vi "Receiver.vi"() -> ()   [LabVIEW 2015]
uses:
  <vilib>/addons/Modulation/Analog/support/mod_Set Error Source.vi
  <vilib>/addons/Modulation/Analog/support/Validators/mod_Fractional Resample Validate.vi
  <vilib>/addons/Modulation/Analog/support/Validators/mod_Check Flush State.vi
  <vilib>/addons/Modulation/Analog/support/mod_FractionalResampler.vi
  <vilib>/addons/Modulation/Analog/support/mod_Integer Rate Interpolation.vi
  <vilib>/addons/Modulation/Analog/support/Validators/mod_Validate Complex Waveform.vi
  <vilib>/addons/Modulation/Analog/support/mod_PerformResampling.vi
  <vilib>/addons/Modulation/Analog/support/Validators/mod_WFErrorHandler.vi
  <vilib>/addons/Modulation/Digital/General/MT Generate PSK System Parameters(M).vi
  <vilib>/addons/Modulation/Digital/Support/Common/Validators/mod_Generate Filter Coefficients Validate.vi
  <vilib>/addons/Modulation/Digital/General/subVIs/mod_Generate Filter Coefficients.vi
  <instrlib>/niUSRP/niUSRP Fetch Rx Data (CDB Cluster).vi
  <vilib>/Utility/error.llb/Error Cluster From Error Code.vi
  <vilib>/addons/Modulation/Analog/support/mod_Resampling Factors.vi
  <vilib>/addons/Modulation/Analog/support/mod_ResamplingFilter.vi
  <vilib>/addons/Modulation/Analog/support/mod_Generate Integer Interpolation Filter.vi
  <vilib>/addons/Modulation/niDMT.lvlib
  <vilib>/addons/Modulation/niAMT.lvlib
panel:
  in  "stop":bool
  in  "Reset":bool=TRUE caption="Reset\nDemodulator?"
  out "measurements":T1={"frequency offset (Hz)"=-11.93165072236316, "frequency drift (Hz)"=0.08770196207837619, "phase offset (deg)"=52.673364140832604} {"phase offset (deg)" format="%.2f"; "frequency drift (Hz)" format="%.2f"; "frequency offset (Hz)" format="%.2f"}
  out "Constellation Graph":T2(graph)
  in  "autoscale":bool
  in  "Acq Duration [sec]":dbl=0.01 format="%#.6p"
  out "Frame Size [samples]":i64=20000
  out "Symbol Rate [Hz]":dbl=125000.0 caption="Symbol Rate, \n[symbols/sec]" format="%.2p"
  in  "filter parameters":T3={"Alpha"=0.5, "Filter Length"=6, "TX Filter"=enum."Root Raised Cos"} {"Alpha" format="%.2f"}
  in  "Choose a PSK Format":enum32{"BPSK", "QPSK"}(tab)=enum."QPSK" caption="PSK"
  in  "BPSK System Parameters":T4={"Samples per Symbol"=8, "symbol map"=[]} {"symbol map" format="%.3f"}
  in  "QPSK System Parameters":T4={"Samples per Symbol"=8, "symbol map"=[]} {"symbol map" format="%.3f"}
  in  "device name":refnum<k15>="192.168.10.4"
  in  "IQ Sampling\nRate [S/sec]":dbl=500000.0 format="%#.6p"
  in  "Carrier\nFrequency [Hz]":dbl=915000000.0 format="%#.6p"
  in  "Gain [dB]":dbl=12.0 format="%#.6p"
  in  "Active Antenna":string(combo)="RX1"
  in  "Enabled Channel":string(combo)="0"
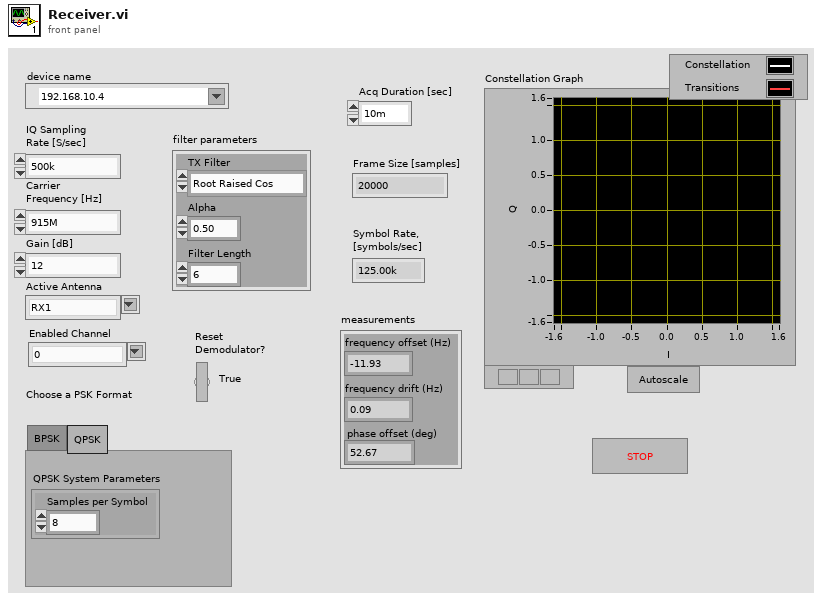
[diagram p1: front panel]
types:
  T1 = cluster{"frequency offset (Hz)":dbl, "frequency drift (Hz)":dbl, "phase offset (deg)":dbl}
  T2 = cluster{"Decimated Array":dbl[], "Decimated Array":dbl[]}[]
  T3 = cluster{"Alpha":dbl, "Filter Length":i32, "TX Filter":enum16{"none", "Raised Cosine", "Root Raised Cos", "Gaussian"}}
  T4 = cluster{"Samples per Symbol":i32, "symbol map":cdb[]}
  T5 = enum16{"none", "Raised Cosine", "Root Raised Cos", "Gaussian"}
  T6 = cluster{"samples per symbol (16)":i32, "symbol map":cdb[], "differential PSK":enum16{"disable", "enable"}, "PSK type":u16}
  T7 = typedef "niAMT.lvlib/Complex Data Waveform.ctl" = cluster{"t0":dbl, "dt":dbl, "Y":cdb[]}
  T8 = cluster{"constellation":dbl[], "oversampled data":dbl[]}[]
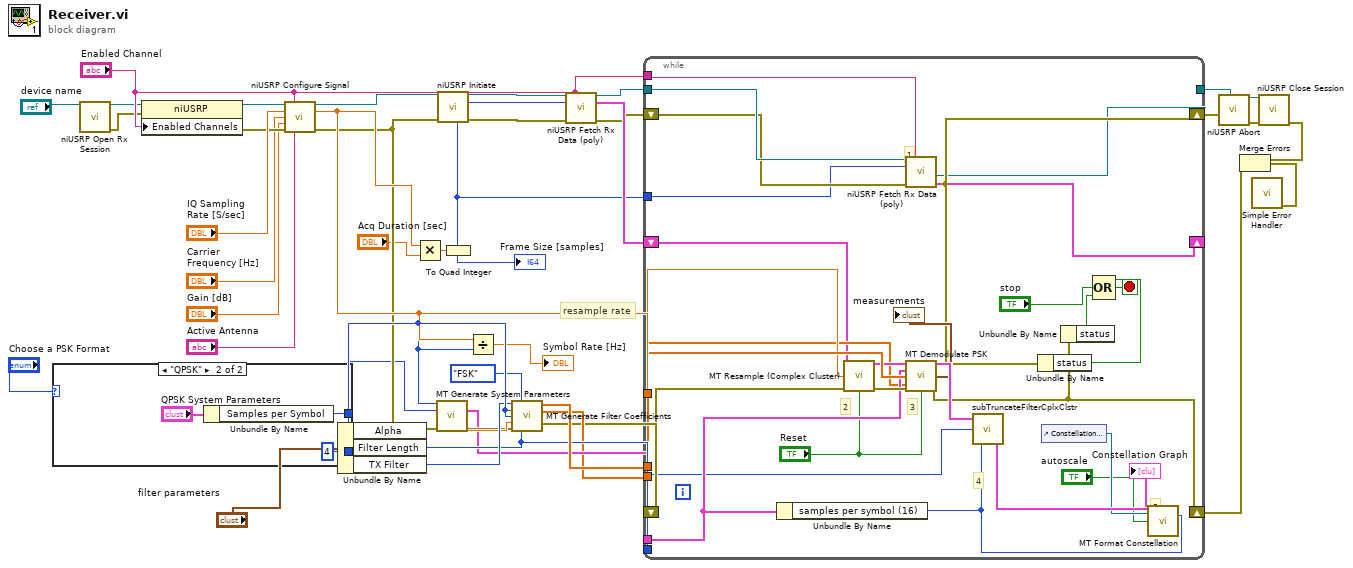
[diagram p0: block diagram]
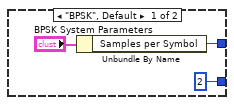
[diagram p2: hidden frame]
diagram:
  # "resample rate"
  n1 = case shown="\"QPSK\"" "Choose a PSK Format" {
    tunnel: [w44 w47] -> w40
    tunnel: [2 ("M-PSK (4)") 4 ("M-PSK (4)")] -> w13
    frame "BPSK", Default {
      n2 = Unbundle By Name("BPSK System Parameters") -> ("Samples per Symbol"=w44:i32)
    }
    frame "QPSK" {
      n3 = Unbundle By Name("QPSK System Parameters") -> ("Samples per Symbol"=w47:i32)
    }
  }
  n4 = call <instrlib>:"niUSRP Open Rx Session.vi"("device names"="device name") -> ("session handle out"=w34:refnum<k15>, "error out"=w35:errorcluster)  [unwired: 13 in]
  n5 = property class="niUSRP"(reference=w34, error in=w35, "Enabled Channels"="Enabled Channel") -> (reference out=w36:refnum<k15>, error out=w37:errorcluster)
  n6 = call <instrlib>:"niUSRP Configure Signal.vi"("session handle"=w36, "channel list"="Enabled Channel", "IQ rate"="IQ Sampling\nRate [S/sec]", "carrier frequency"="Carrier\nFrequency [Hz]", "gain"="Gain [dB]", "error in (no error)"=w37, "active antenna"="Active Antenna") -> ("session handle out"=w24:refnum<k15>, "coerced IQ rate"=w42:dbl, "error out"=w25:errorcluster)  [unwired: 4 in, 2 out]
  n7 = Unbundle By Name("filter parameters") -> ("Alpha"=w10:dbl, "Filter Length"=w11:i32, "TX Filter"=w12:T5)
  n8 = Multiply(x=w42, y="Acq Duration [sec]") -> (x*y=w3:dbl)
  n9 = call-poly <vilib>:"MT Generate System Parameters.vi"("samples per symbol (16)"=w40, "M-PSK (4)"=w13, "error in (no error)"=w25) -> ("PSK system parameters"=w7:T6, "error out"=w8:errorcluster)  [unwired: 10 in, 1 out]
  n10 = call <instrlib>:"niUSRP Initiate.vi"("session handle"=w24, "error in (no error)"=w25) -> ("session handle out"=w26:refnum<k15>, "error out"=w27:errorcluster)  [unwired: 12 in]
  n11 = To Quad Integer(1:w3) -> (0:w28:i64)
  "Frame Size [samples]" <- w28
  n12 = Divide(x=w42, y=w40) -> (x/y=→"Symbol Rate [Hz]":dbl)
  n13 = call <vilib>:"MT Generate Filter Coefficients.vi"("pulse shaping filter (none)"=w12, "modulation type"=enum16{"FSK", "PSK"}."FSK", "pulse shaping samples per symbol (16)"=w40, "matched samples per symbol (16)"=w40, "filter parameter"=w10, "error in (no error)"=w8, "filter length (symbols)"=w11) -> ("pulse shaping filter coefficients"=w15:dbl[], "matched filter coefficients"=w6:dbl[], "error out"=w5:errorcluster)  [unwired: 6 in]
  n14 = call-poly <instrlib>:"niUSRP Fetch Rx Data (poly).vi"("session handle"=w26, "channel list"="Enabled Channel", "number of samples"=w28, "error in (no error)"=w27) -> ("session handle out"=w30:refnum<k15>, "data"=w31:cluster{"t0":dbl, "dt":dbl, "Y":cdb[]}, "error out"=w29:errorcluster)  [unwired: 8 in, 1 out]
  n15 = while {
    tunnel: [w49] -> w19
    shift-right: [w51] -> w18
    shift-left: w29 -> [w55]
    shift-right: [w65] -> w33
    shift-left: w5 -> [w66]
    tunnel: w28 -> [w54]
    tunnel: w30 -> [w56]
    tunnel: w6 -> [w75]
    tunnel: w7 -> [w71]
    tunnel: w42 -> [w72]
    tunnel: w11 -> [w70]
    tunnel: w15 -> [w62]
    shift-right: [w52] -> _
    shift-left: w31 -> [w53]
    tunnel: "Enabled Channel" -> [w50]
    stop <- w77 stop-if-true
    # "5"
    # "4"
    # "3"
    # "2"
    # "1"
    n16 = Unbundle By Name(w71) -> ("samples per symbol (16)"=w67:i32)
    n17 = call <vilib>:"MT Resample (Complex Cluster).vi"("input complex waveform"=w53, "desired sample rate (Hz)"=w72, "error in (no error)"=w66, "reset? (T)"="Reset") -> ("output complex waveform"=w74:T7, "error out"=w73:errorcluster)  [unwired: 10 in]
    n18 = call-poly <instrlib>:"niUSRP Fetch Rx Data (poly).vi"("session handle"=w56, "channel list"=w50, "number of samples"=w54, "error in (no error)"=w55) -> ("session handle out"=w49:refnum<k15>, "data"=w52:cluster{"t0":dbl, "dt":dbl, "Y":cdb[]}, "error out"=w51:errorcluster)  [unwired: 8 in, 1 out]
    n19 = call <vilib>:"MT Demodulate PSK.vi"("input complex waveform"=w74, "PSK system parameters"=w71, "matched filter coefficients"=w75, "error in (no error)"=w73, "pulse shaping filter coefficients"=w62, "reset? (T)"="Reset") -> ("recovered complex waveform"=w69:T7, "measurements"=→"measurements":T1, "error out"=w65:errorcluster)  [unwired: 5 in, 2 out]
    n20 = call "subTruncateFilterCplxClstr.vi"("samples per symbol (16)"=w67, "filter length (symbols)"=w70, "waveform to truncate"=w69) -> ("truncated waveform"=w68:T7)
    n21 = Unbundle By Name(w51) -> ("status"=w76:bool)
    n22 = control-ref of="Constellation Graph"() -> (w60:refnum<vi>)
    n23 = Unbundle By Name(w65) -> ("status"=w63:bool)
    n24 = Compound Arithmetic op=OR(w76, "stop", w63) -> (w77:bool)
    n25 = call <vilib>:"MT Format Constellation.vi"("waveform"=w68, "constellation reference"=w60, "samples per symbol"=w67, "autoscale"="autoscale") -> ("constellation graph"=→"Constellation Graph":T8)  [unwired: 10 in, 1 out]
  }
  n26 = call <instrlib>:"niUSRP Abort.vi"("session handle"=w19, "error in (no error)"=w18) -> ("session handle out"=w16:refnum<k15>, "error out"=w17:errorcluster)  [unwired: 12 in]
  n27 = call <instrlib>:"niUSRP Close Session.vi"("session handle"=w16, "error in (no error)"=w17) -> ("error out"=w32:errorcluster)  [unwired: 13 in]
  n28 = Merge Errors(w32, w33) -> (w1:errorcluster)
  n29 = call <vilib>:"Simple Error Handler.vi"("error in (no error)"=w1) -> ()  [unwired: 4 in, 5 out]
